vi "GetAllControlRefs_Path.vi"(4 "Add Array Ctls?":bool=TRUE, 6 "Add Cluster Ctls?":bool=TRUE, 8 "error in (no error)":errorcluster, 11 "VI Path":path) -> (0 "error out":errorcluster, 3 "CtlLookup out":T1)   [LabVIEW 2020, in "CtlReferences.lvlib" / "CtlReferences.lvclass"]
doc: "generate all of the Control Refs for a give VI"
uses:
  CtlReferences.lvclass
  CtlReferences.lvclass/CtlReferences.ctl
  TypeDefs/CtlLookup.ctl
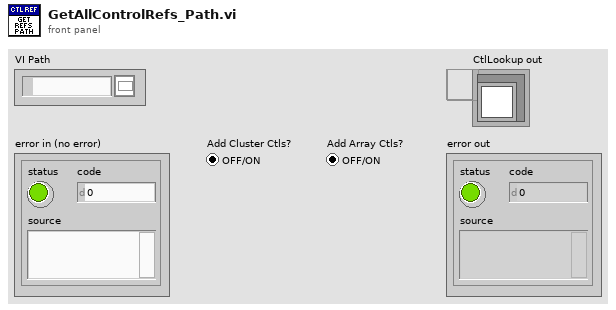
[diagram p1: front panel]
types:
  T1 = typedef "CtlReferences.lvlib/CtlReferences.lvclass/CtlLookup.ctl" = refnum<data-value>
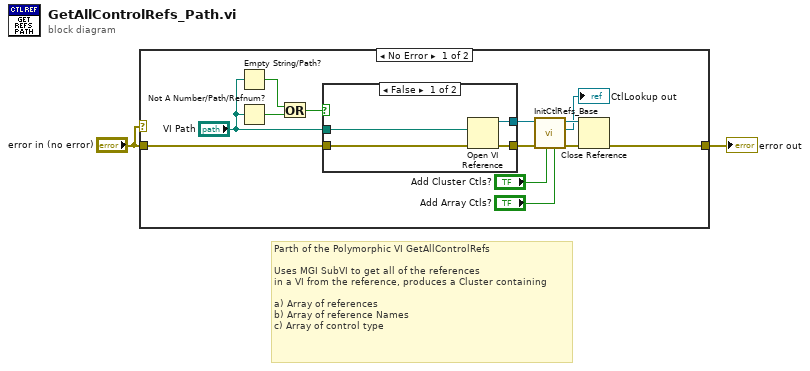
[diagram p0: block diagram]
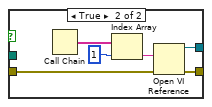
[diagram p2: hidden frame]
diagram:
  # "Parth of the Polymorphic VI GetAllControlRefs\n\nUses MGI SubVI to get all of the references \nin a VI from the reference, produces a Cluster containing\n\na) Array of references\nb) Array of reference Names\nc) Array of control type"
  n1 = case shown="No Error" "error in (no error)" {
    tunnel: [w10 w26] -> w2
    tunnel: "error in (no error)" -> [w15 w26]
    frame No Error {
      n2 = Empty String/Path?(string/path="VI Path") -> (empty?=w13:bool)
      n3 = Not A Number/Path/Refnum?(number/path/refnum="VI Path") -> (NaN/Path/Refnum?=w12:bool)
      n4 = Or(x=w13, y=w12) -> (x .or. y?=w11:bool)
      n5 = case shown="False" w11 {
        tunnel: w15 -> [w17 w20]
        tunnel: [w18 w22] -> w9
        tunnel: "VI Path" -> [w16 _]
        tunnel: [w19 w21] -> w8
        frame False {
          n6 = Open VI Reference(vi path=w16, error in (no error)=w17) -> (vi reference=w19:refnum<vi>, error out=w18:errorcluster)  [unwired: 4 in]
        }
        frame True {
          n7 = Call Chain() -> (call chain=w24:string[])
          n8 = Index Array(array=w24, index=1) -> (element=w23:string)
          n9 = Open VI Reference(vi path=w23, error in (no error)=w20) -> (vi reference=w21:refnum<vi>, error out=w22:errorcluster)  [unwired: 4 in]
        }
      }
      n10 = call "InitCtlRefs_Base.vi"("Add Array Ctls?"="Add Array Ctls?", "Add Cluster Ctls?"="Add Cluster Ctls?", "error in (no error)"=w9, "VI in"=w8) -> ("error out"=w5:errorcluster, "Data Value Reference out"=→"CtlLookup out":T1, "VI out"=w7:refnum<vi>)  [unwired: 5 in]
      n11 = Close Reference(reference=w7, error in (no error)=w5) -> (error out=w10:errorcluster)
    }
    frame Error {
    }
  }
  "error out" <- w2
